vi "Boolean Calculator.vi"() -> ()   [LabVIEW 2009]
panel:
  out "Boolean 3":bool
  in  "Boolean 2":bool
  in  "Boolean":bool
  in  "Combo Box":string(combo)
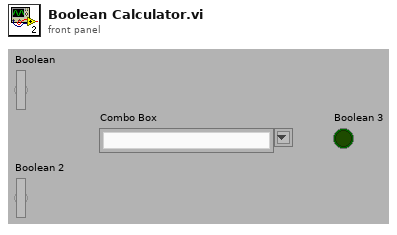
[diagram p1: front panel]
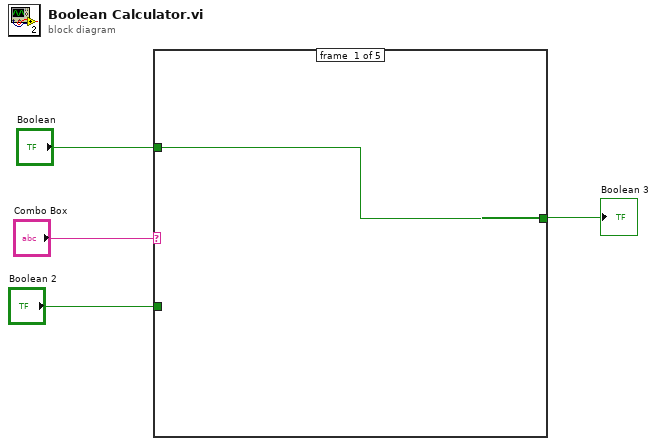
[diagram p0: block diagram]
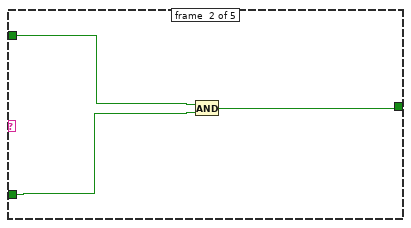
[diagram p2: hidden frame]
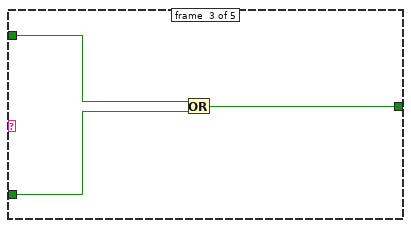
[diagram p3: hidden frame]
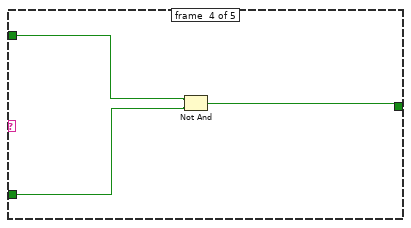
[diagram p4: hidden frame]
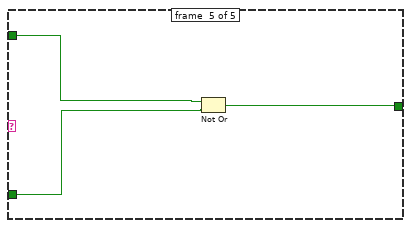
[diagram p5: hidden frame]
diagram:
  n1 = case shown="\"AND\"" "Combo Box" {
    tunnel: [w5 w6 w9 w14 w17] -> w1
    tunnel: "Boolean" -> [w5 w8 w10 w13 w16]
    tunnel: "Boolean 2" -> [_ w7 w11 w12 w15]
    frame #0 {
    }
    frame #1 {
      n2 = And(x=w8, y=w7) -> (x .and. y?=w6:bool)
    }
    frame #2 {
      n3 = Or(x=w10, y=w11) -> (x .or. y?=w9:bool)
    }
    frame #3 {
      n4 = Not And(1:w12, 2:w13) -> (0:w14:bool)
    }
    frame #4 {
      n5 = Not Or(1:w15, 2:w16) -> (0:w17:bool)
    }
  }
  "Boolean 3" <- w1
